vi "Subscriber1.vi"() -> ()   [LabVIEW 2021]
uses:
  ChannelCommon/typedef/Datatype Waveform.ctl
  CIFChannels/Typedef/Direction.ctl
  ChannelCommon/typedef/FIFO Config.ctl
  CIF_NIChn/FIFO_DAQ/CIF_NIChn_Fifo_DAQ.lvclass
  <vilib>/CIF Foundation/CIF Utilities/DataTypes/Flatten U64.vi
  ChannelCommon/ChannelCommon.lvlib
  CIFChannels/CIFChannels.lvclass
panel:
  out "DAQ Out":T1[](array[typedef])
  in  "stop":bool
  in  "Publisher":string
  out "pass":bool
  out "error out":errorcluster
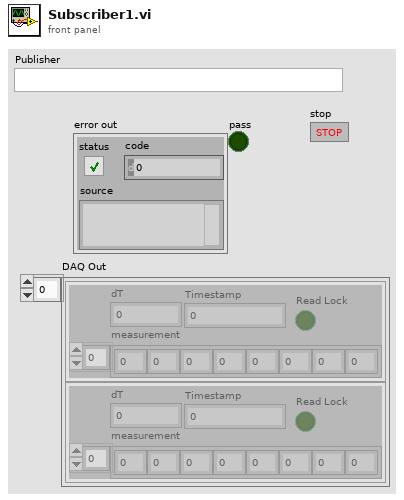
[diagram p1: front panel]
types:
  T1 = typedef "ChannelCommon.lvlib/Datatype Waveform.ctl" = cluster{"measurement":dbl[], "dT":dbl, "Timestamp":i64, "Read Lock":bool}
  T2 = typedef "ChannelCommon.lvlib/FIFO Config.ctl" = cluster{"Max Bytes/Msg":u64, "Max Msg/FIFO":u64, "Flags":u64}
  T3 = typedef "CIFChannels.lvclass/Direction.ctl" = enum16{"Publisher", "Subscriber"}
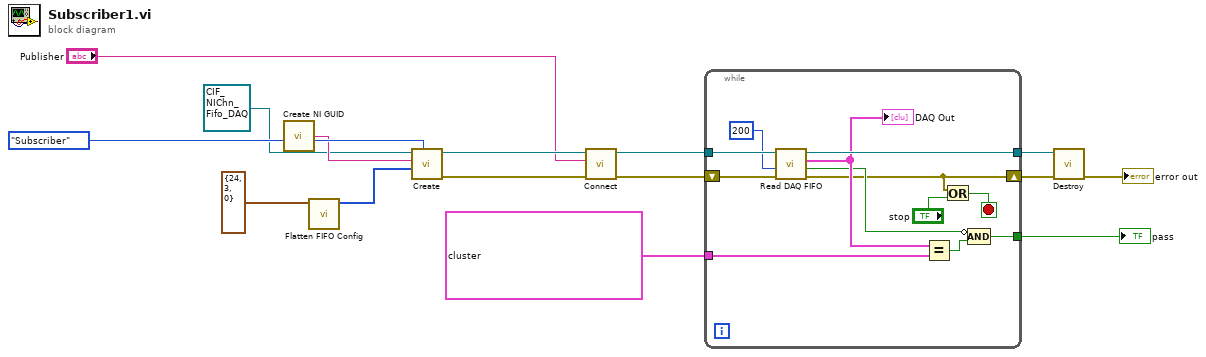
[diagram p0: block diagram]
diagram:
  n1 = call <vilib>:"Create NI GUID.vi"() -> ("NI GUID"=w12:string)
  n2 = call "Flatten FIFO Config.vi"("FIFO Config in"=T2 {"Max Bytes/Msg"=24, "Max Msg/FIFO"=3, "Flags"=0}) -> ("Flattened FIFO Config"=w6:u8[])  [unwired: 10 in]
  n3 = call-dynamic "Create.vi"("Direction"=Direction."Subscriber", "Custom Config Data"=w6, "Name"=w12, "CIFFIFO in"=refnum<class "CIF_NIChn_Fifo_DAQ.lvclass"> refnum ("CIF_NIChn_Fifo_Power.lvclass")) -> ("error out"=w10:errorcluster, "CIFFIFO out"=w9:refnum<class "CIF_NIChn_Fifo_DAQ.lvclass">)  [unwired: 6 in]
  n4 = call-dynamic "Connect.vi"("error in (no error)"=w10, "Connection Name"="Publisher", "CIFTag in"=w9) -> ("error out"=w2:errorcluster, "CIFTag out"=w8:refnum<class "CIF_NIChn_Fifo_DAQ.lvclass">)  [unwired: 7 in]
  n5 = while {
    tunnel: [w27] -> w14
    tunnel: w8 -> [w25]
    tunnel: T1[] [{"measurement"=array[986 elements], "dT"=43.0, "Timestamp"=2, "Read Lock"=FALSE}, {"measurement"=array[1001 elements], "dT"=34.0, "Timestamp"=1, "Read Lock"=FALSE}] ("DAQ In") -> [w21]
    tunnel: [w20] -> w5
    shift-right: [w18] -> w1
    shift-left: w2 -> [w19]
    stop <- w16 stop-if-true
    n6 = call-dynamic "Read DAQ FIFO.vi"("error in (no error)"=w19, "Timeout (ms)"=200, "CIF_NIChn_FIFO_DAQ in"=w25) -> ("error out"=w18:errorcluster, "timed out?"=w23:bool, "Data Out"=w24:T1[], "CIF_NIChn_FIFO_DAQ out"=w27:refnum<class "CIF_NIChn_Fifo_DAQ.lvclass">)  [unwired: 4 in, 1 out]
    "DAQ Out" <- w24
    n7 = Equal?(x=w24, y=w21) -> (x = y?=w26:bool)
    n8 = Or(x=w18, y="stop") -> (x .or. y?=w16:bool)
    n9 = Compound Arithmetic op=AND(invert w23, w26) -> (w20:bool)
  }
  "pass" <- w5
  n10 = call-dynamic "Destroy.vi"("error in (no error)"=w1, "CIFFIFO in"=w14) -> ("error out"=→"error out":errorcluster)  [unwired: 8 in, 1 out]
